vi "CalcDifferences.vi"(8 "error in (no error)":errorcluster, 10 "PointsIn (pixels)":dbl[][](array[numeric]), 11 "Iterations":i32=2) -> (0 "error out":errorcluster, 3 "Differences":dbl)   [LabVIEW 2010]
uses:
  <vilib>/Analysis/_algsub.llb/Real Vector Norm.vi
  <vilib>/Analysis/NI_AALPro.lvlib
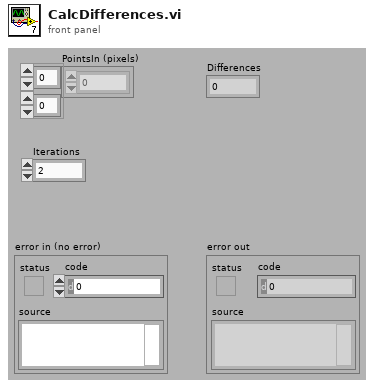
[diagram p1: front panel]
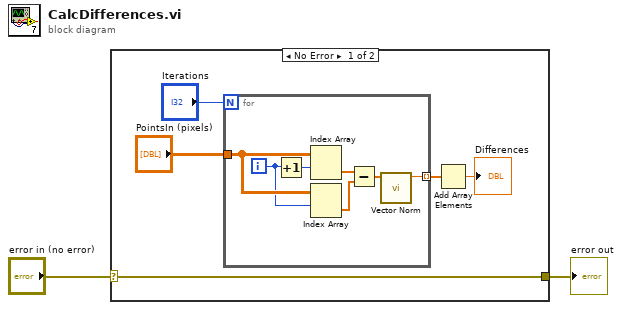
[diagram p0: block diagram]
diagram:
  n1 = case shown="No Error" "error in (no error)" {
    selector: "error in (no error)" -> [w3 w15]
    tunnel: [w3 w15] -> w1
    frame No Error {
      n2 = for {
        N: "Iterations" -> [_]
        tunnel: "PointsIn (pixels)" -> [w14]
        tunnel: [w8] -> w6 mode=indexing
        i -> [w12]
        n3 = Increment(x=w12) -> (x+1=w13:i32)
        n4 = Index Array(array=w14, index (row)=w13) -> (element=w11:dbl[])  [unwired: 1 in]
        n5 = Index Array(array=w14, index (row)=w12) -> (element=w10:dbl[])  [unwired: 1 in]
        n6 = Subtract(x=w11, y=w10) -> (x-y=w9:dbl[])
        n7 = call-poly <vilib>:"Vector Norm.vi"("Input Vector"=w9) -> ("norm"=w8:dbl)  [unwired: 9 in, 1 out]
      }
      n8 = Add Array Elements(numeric array=w6) -> (sum=→"Differences":dbl)
    }
    frame Error {
    }
  }
  "error out" <- w1
